vi "测试报告_表格.vi"() -> ()   [LabVIEW 2010]
uses:
  <vilib>/Utility/NIReport.llb/NI_report.lvclass
  全局量/自动测试结果.vi
  <vilib>/Utility/NIReport.llb/Append Report Text (str wrap).vi
panel:
  out "XY图":cluster{"Y":dbl[], "Y":dbl[]}[](graph)
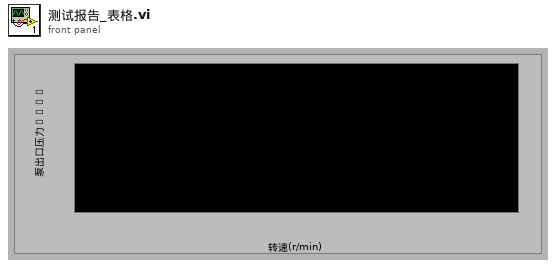
[diagram p1: front panel]
types:
  T1 = enum16{"maximized", "minimized", "normal", "no change"}
  T2 = enum16{"Standard Report", "HTML", "Word", "Excel"}
  T3 = cluster{"position (excel)":cluster{"row":i32, "column":i32}, "name (excel)":string, string}
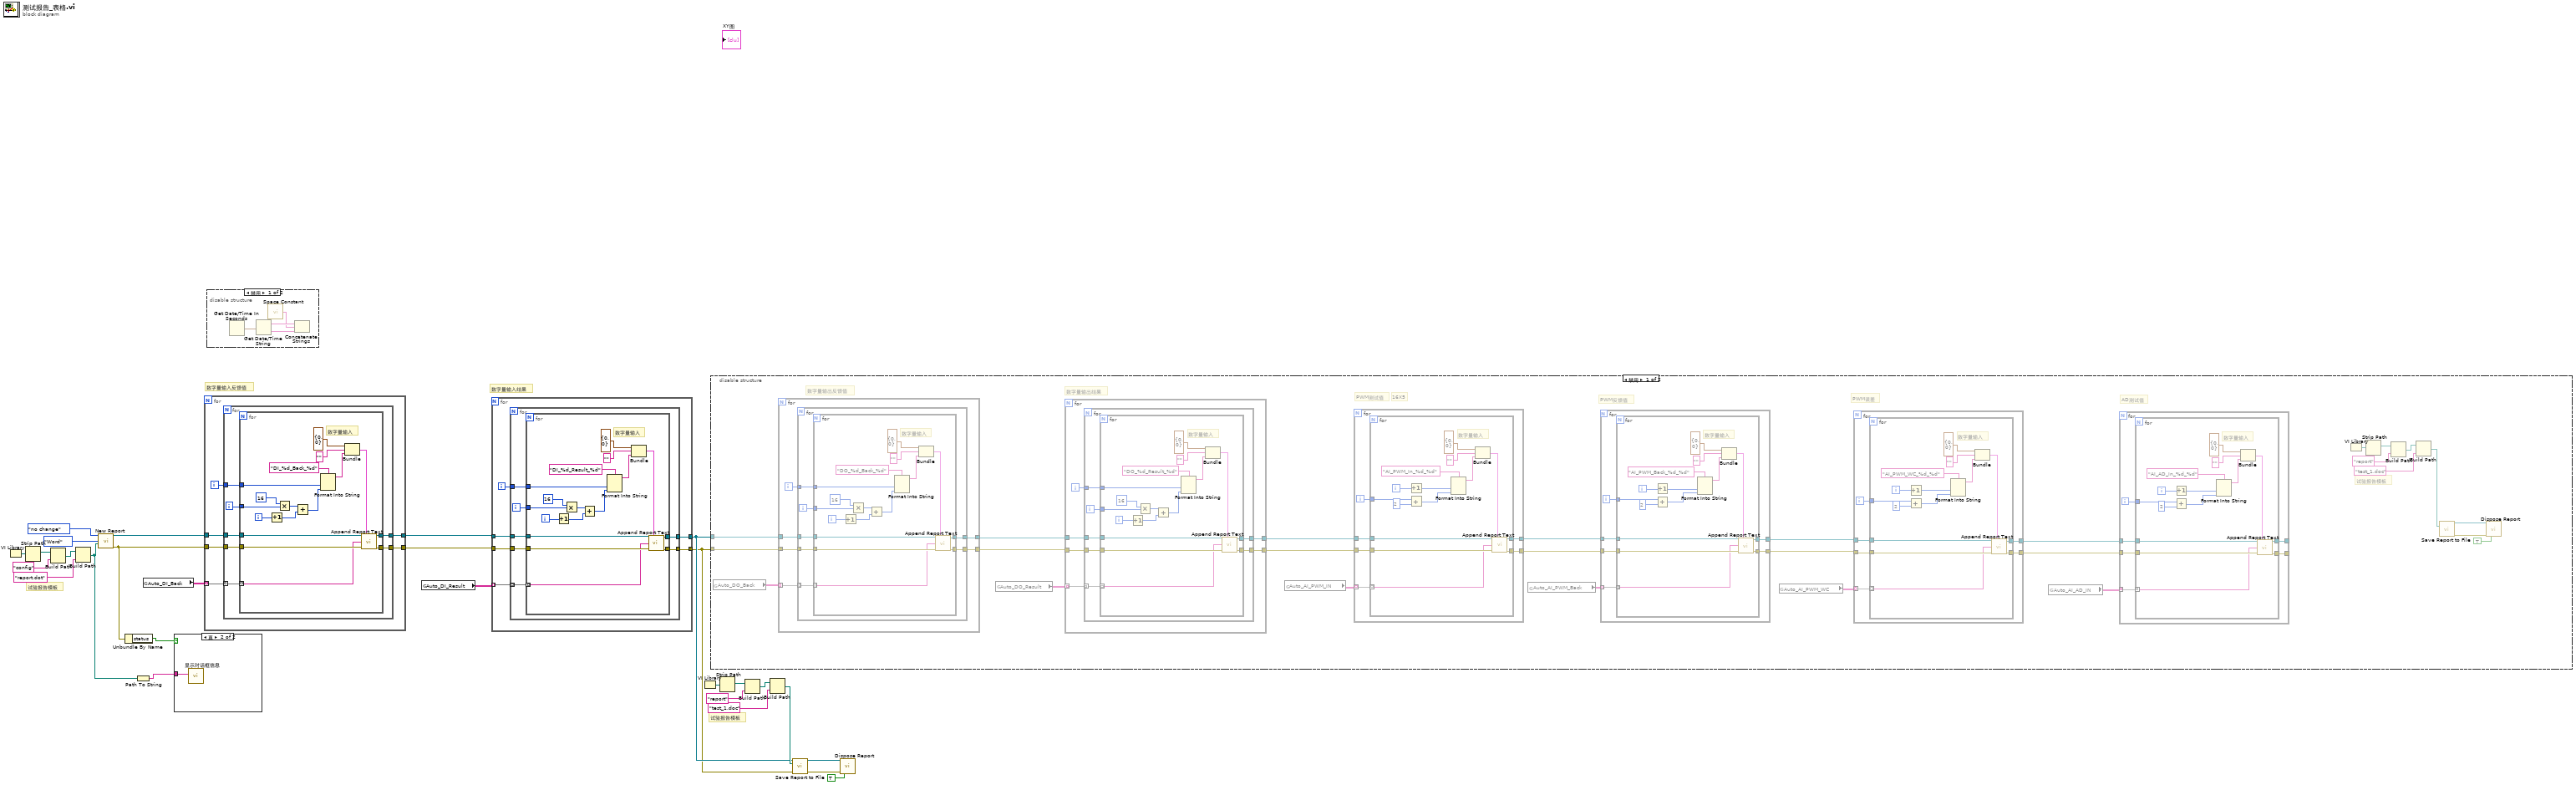
[diagram p0: block diagram]
diagram:
  # "试验报告模板"
  # "数字量输入结果"
  # "数字量输入反馈值"
  # "试验报告模板"
  n1 = VI Library() -> (path=w23:path)
  n2 = Strip Path(path=w23) -> (stripped path=w26:path)  [unwired: 1 out]
  n3 = Build Path(base path=w26, name or relative path="config") -> (appended path=w24:path)
  n4 = Build Path(base path=w24, name or relative path="report.dot") -> (appended path=w2:path)
  n5 = call <vilib>:"New Report.vi"("window state (normal)"=T1."no change", "report type"=T2."Word", "template (empty)"=w2) -> ("report out"=w21:refnum<class "NI_report.lvclass">, "error out"=w5:errorcluster)  [unwired: 11 in]
  n6 = Unbundle By Name(w5) -> ("status"=w4:bool)
  n7 = Path To String(path=w2) -> (string=w1:string)
  n8 = global read "自动测试结果.vi" "Auto_DI_Back"() -> (w20:string[][][])
  n9 = case shown="真" w4 {
    tunnel: w1 -> [_ w28]
    frame False {
    }
    frame True {
      n10 = call "显示对话框信息"("Message"=w28) -> ()  [unwired: 9 in, 2 out]
    }
  }
  n11 = for {
    tunnel: w21 -> [w34]
    tunnel: w5 -> [w33]
    tunnel: [w32] -> w19
    tunnel: [w31] -> w18
    tunnel: w20 -> [w30] mode=indexing
    i -> [w29]
    n12 = for {
      tunnel: w34 -> [w41]
      tunnel: w33 -> [w40]
      tunnel: [w39] -> w32
      tunnel: [w38] -> w31
      tunnel: w30 -> [w36] mode=indexing
      tunnel: w29 -> [w35]
      i -> [w37]
      n13 = for {
        tunnel: w41 -> [w58]
        tunnel: w40 -> [w57]
        tunnel: [w55] -> w39
        tunnel: [w54] -> w38
        tunnel: w37 -> [w46]
        tunnel: w36 -> [w44] mode=indexing
        tunnel: w35 -> [w43]
        i -> [w45]
        # "数字量输入"
        n14 = Increment(x=w45) -> (x+1=w47:i32)
        n15 = Multiply(x=16, y=w46) -> (x*y=w48:i32)
        n16 = Add(x=w48, y=w47) -> (x+y=w42:i32)
        n17 = Format Into String(format string="DI_%d_Back_%d" ("bookmark (word)"), w43, w42) -> (resulting string=w51:string)  [unwired: 2 in, 1 out]
        n18 = Bundle("position (excel)"=cluster{"row":i32, "column":i32} {"row"=0, "column"=0}, "name (excel)"="", w51) -> (w50:T3)  [unwired: 1 in]
        n19 = call-poly <vilib>:"Append Report Text.vi"("report in"=w58, "MS Office parameters"=w50, "text"=w44, "error in (no error)"=w57) -> ("report out"=w55:refnum<class "NI_report.lvclass">, "error out"=w54:errorcluster)  [unwired: 8 in, 2 out]
      }
    }
  }
  n20 = disable-structure shown="禁用" {
    frame Disabled {
      n21 = Get Date/Time In Seconds() -> (seconds since 1Jan1904=w62:timestamp)
      n22 = Get Date/Time String(seconds (now)=w62) -> (date string=w61:string, time string=w60:string)  [unwired: 2 in]
      n23 = call <vilib>:"Space Constant.vi"() -> ("String"=w59:string)
      n24 = Concatenate Strings(w61, w59, w60) -> ()  [unwired: 1 out]
    }
    frame Enabled {
    }
  }
  n25 = global read "自动测试结果.vi" "Auto_DI_Result"() -> (w17:string[][][])
  n26 = for {
    tunnel: w19 -> [w68]
    tunnel: w18 -> [w67]
    tunnel: [w66] -> w7
    tunnel: [w65] -> w6
    tunnel: w17 -> [w64] mode=indexing
    i -> [w63]
    n27 = for {
      tunnel: w68 -> [w75]
      tunnel: w67 -> [w74]
      tunnel: [w73] -> w66
      tunnel: [w72] -> w65
      tunnel: w64 -> [w70] mode=indexing
      tunnel: w63 -> [w69]
      i -> [w71]
      n28 = for {
        tunnel: w75 -> [w92]
        tunnel: w74 -> [w91]
        tunnel: [w89] -> w73
        tunnel: [w88] -> w72
        tunnel: w71 -> [w80]
        tunnel: w70 -> [w78] mode=indexing
        tunnel: w69 -> [w77]
        i -> [w79]
        # "数字量输入"
        n29 = Increment(x=w79) -> (x+1=w81:i32)
        n30 = Multiply(x=16, y=w80) -> (x*y=w82:i32)
        n31 = Add(x=w82, y=w81) -> (x+y=w76:i32)
        n32 = Format Into String(format string="DI_%d_Result_%d" ("bookmark (word)"), w77, w76) -> (resulting string=w85:string)  [unwired: 2 in, 1 out]
        n33 = Bundle("position (excel)"=cluster{"row":i32, "column":i32} {"row"=0, "column"=0}, "name (excel)"="", w85) -> (w84:T3)  [unwired: 1 in]
        n34 = call-poly <vilib>:"Append Report Text.vi"("report in"=w92, "MS Office parameters"=w84, "text"=w78, "error in (no error)"=w91) -> ("report out"=w89:refnum<class "NI_report.lvclass">, "error out"=w88:errorcluster)  [unwired: 8 in, 2 out]
      }
    }
  }
  n35 = VI Library() -> (path=w8:path)
  n36 = disable-structure shown="禁用" {
    disable-tunnel: w7 -> [w110 _]
    disable-tunnel: w6 -> [w109 _]
    frame Disabled {
      # "AD测试值"
      # "PWM误差"
      # "PWM反馈值"
      # "16X5"
      # "PWM测试值"
      # "数字量输出结果"
      # "数字量输出反馈值"
      # "试验报告模板"
      n37 = global read "自动测试结果.vi" "Auto_DO_Back"() -> (w108:string[][][])
      n38 = for {
        tunnel: w110 -> [w239]
        tunnel: w109 -> [w238]
        tunnel: [w237] -> w106
        tunnel: [w236] -> w105
        tunnel: w108 -> [w235] mode=indexing
        i -> [w234]
        n39 = for {
          tunnel: w239 -> [w246]
          tunnel: w238 -> [w245]
          tunnel: [w244] -> w237
          tunnel: [w243] -> w236
          tunnel: w235 -> [w241] mode=indexing
          tunnel: w234 -> [w240]
          i -> [w242]
          n40 = for {
            tunnel: w246 -> [w263]
            tunnel: w245 -> [w262]
            tunnel: [w260] -> w244
            tunnel: [w259] -> w243
            tunnel: w242 -> [w251]
            tunnel: w241 -> [w249] mode=indexing
            tunnel: w240 -> [w248]
            i -> [w250]
            # "数字量输入"
            n41 = Increment(x=w250) -> (x+1=w252:i32)
            n42 = Multiply(x=16, y=w251) -> (x*y=w253:i32)
            n43 = Add(x=w253, y=w252) -> (x+y=w247:i32)
            n44 = Format Into String(format string="DO_%d_Back_%d" ("bookmark (word)"), w248, w247) -> (resulting string=w256:string)  [unwired: 2 in, 1 out]
            n45 = Bundle("position (excel)"=cluster{"row":i32, "column":i32} {"row"=0, "column"=0}, "name (excel)"="", w256) -> (w255:T3)  [unwired: 1 in]
            n46 = call-poly <vilib>:"Append Report Text.vi"("report in"=w263, "MS Office parameters"=w255, "text"=w249, "error in (no error)"=w262) -> ("report out"=w260:refnum<class "NI_report.lvclass">, "error out"=w259:errorcluster)  [unwired: 8 in, 2 out]
          }
        }
      }
      n47 = global read "自动测试结果.vi" "Auto_DO_Result"() -> (w107:string[][][])
      n48 = for {
        tunnel: w106 -> [w209]
        tunnel: w105 -> [w208]
        tunnel: [w207] -> w103
        tunnel: [w206] -> w102
        tunnel: w107 -> [w205] mode=indexing
        i -> [w204]
        n49 = for {
          tunnel: w209 -> [w216]
          tunnel: w208 -> [w215]
          tunnel: [w214] -> w207
          tunnel: [w213] -> w206
          tunnel: w205 -> [w211] mode=indexing
          tunnel: w204 -> [w210]
          i -> [w212]
          n50 = for {
            tunnel: w216 -> [w233]
            tunnel: w215 -> [w232]
            tunnel: [w230] -> w214
            tunnel: [w229] -> w213
            tunnel: w212 -> [w221]
            tunnel: w211 -> [w219] mode=indexing
            tunnel: w210 -> [w218]
            i -> [w220]
            # "数字量输入"
            n51 = Increment(x=w220) -> (x+1=w222:i32)
            n52 = Multiply(x=16, y=w221) -> (x*y=w223:i32)
            n53 = Add(x=w223, y=w222) -> (x+y=w217:i32)
            n54 = Format Into String(format string="DO_%d_Result_%d" ("bookmark (word)"), w218, w217) -> (resulting string=w226:string)  [unwired: 2 in, 1 out]
            n55 = Bundle("position (excel)"=cluster{"row":i32, "column":i32} {"row"=0, "column"=0}, "name (excel)"="", w226) -> (w225:T3)  [unwired: 1 in]
            n56 = call-poly <vilib>:"Append Report Text.vi"("report in"=w233, "MS Office parameters"=w225, "text"=w219, "error in (no error)"=w232) -> ("report out"=w230:refnum<class "NI_report.lvclass">, "error out"=w229:errorcluster)  [unwired: 8 in, 2 out]
          }
        }
      }
      n57 = global read "自动测试结果.vi" "Auto_AI_PWM_IN"() -> (w104:string[][])
      n58 = for {
        tunnel: w103 -> [w188]
        tunnel: w102 -> [w187]
        tunnel: [w186] -> w100
        tunnel: [w185] -> w99
        tunnel: w104 -> [w184] mode=indexing
        i -> [w183]
        n59 = for {
          tunnel: w188 -> [w203]
          tunnel: w187 -> [w202]
          tunnel: [w200] -> w186
          tunnel: [w199] -> w185
          tunnel: w184 -> [w194] mode=indexing
          tunnel: w183 -> [w191]
          i -> [w193]
          # "数字量输入"
          n60 = Increment(x=w193) -> (x+1=w192:i32)
          n61 = Add(x=w191, y=2) -> (x+y=w189:i32)
          n62 = Format Into String(format string="AI_PWM_In_%d_%d" ("bookmark (word)"), w192, w189) -> (resulting string=w196:string)  [unwired: 2 in, 1 out]
          n63 = Bundle("position (excel)"=cluster{"row":i32, "column":i32} {"row"=0, "column"=0}, "name (excel)"="", w196) -> (w195:T3)  [unwired: 1 in]
          n64 = call-poly <vilib>:"Append Report Text.vi"("report in"=w203, "MS Office parameters"=w195, "text"=w194, "error in (no error)"=w202) -> ("report out"=w200:refnum<class "NI_report.lvclass">, "error out"=w199:errorcluster)  [unwired: 8 in, 2 out]
        }
      }
      n65 = global read "自动测试结果.vi" "Auto_AI_PWM_Back"() -> (w101:string[][])
      n66 = for {
        tunnel: w100 -> [w167]
        tunnel: w99 -> [w166]
        tunnel: [w165] -> w97
        tunnel: [w164] -> w96
        tunnel: w101 -> [w163] mode=indexing
        i -> [w162]
        n67 = for {
          tunnel: w167 -> [w182]
          tunnel: w166 -> [w181]
          tunnel: [w179] -> w165
          tunnel: [w178] -> w164
          tunnel: w163 -> [w173] mode=indexing
          tunnel: w162 -> [w170]
          i -> [w172]
          # "数字量输入"
          n68 = Increment(x=w172) -> (x+1=w171:i32)
          n69 = Add(x=w170, y=2) -> (x+y=w168:i32)
          n70 = Format Into String(format string="AI_PWM_Back_%d_%d" ("bookmark (word)"), w171, w168) -> (resulting string=w175:string)  [unwired: 2 in, 1 out]
          n71 = Bundle("position (excel)"=cluster{"row":i32, "column":i32} {"row"=0, "column"=0}, "name (excel)"="", w175) -> (w174:T3)  [unwired: 1 in]
          n72 = call-poly <vilib>:"Append Report Text.vi"("report in"=w182, "MS Office parameters"=w174, "text"=w173, "error in (no error)"=w181) -> ("report out"=w179:refnum<class "NI_report.lvclass">, "error out"=w178:errorcluster)  [unwired: 8 in, 2 out]
        }
      }
      n73 = global read "自动测试结果.vi" "Auto_AI_PWM_WC"() -> (w98:string[][])
      n74 = for {
        tunnel: w97 -> [w146]
        tunnel: w96 -> [w145]
        tunnel: [w144] -> w95
        tunnel: [w143] -> w94
        tunnel: w98 -> [w141] mode=indexing
        i -> [w142]
        n75 = for {
          tunnel: w146 -> [w161]
          tunnel: w145 -> [w160]
          tunnel: [w158] -> w144
          tunnel: [w157] -> w143
          tunnel: w141 -> [w152] mode=indexing
          tunnel: w142 -> [w149]
          i -> [w151]
          # "数字量输入"
          n76 = Increment(x=w151) -> (x+1=w150:i32)
          n77 = Add(x=w149, y=2) -> (x+y=w147:i32)
          n78 = Format Into String(format string="AI_PWM_WC_%d_%d" ("bookmark (word)"), w150, w147) -> (resulting string=w154:string)  [unwired: 2 in, 1 out]
          n79 = Bundle("position (excel)"=cluster{"row":i32, "column":i32} {"row"=0, "column"=0}, "name (excel)"="", w154) -> (w153:T3)  [unwired: 1 in]
          n80 = call-poly <vilib>:"Append Report Text.vi"("report in"=w161, "MS Office parameters"=w153, "text"=w152, "error in (no error)"=w160) -> ("report out"=w158:refnum<class "NI_report.lvclass">, "error out"=w157:errorcluster)  [unwired: 8 in, 2 out]
        }
      }
      n81 = global read "自动测试结果.vi" "Auto_AI_AD_IN"() -> (w93:string[][])
      n82 = for {
        tunnel: w95 -> [w125]
        tunnel: w94 -> [w124]
        tunnel: [w123] -> _
        tunnel: [w122] -> _
        tunnel: w93 -> [w120] mode=indexing
        i -> [w121]
        n83 = for {
          tunnel: w125 -> [w140]
          tunnel: w124 -> [w139]
          tunnel: [w137] -> w123
          tunnel: [w136] -> w122
          tunnel: w120 -> [w131] mode=indexing
          tunnel: w121 -> [w128]
          i -> [w130]
          # "数字量输入"
          n84 = Increment(x=w130) -> (x+1=w129:i32)
          n85 = Add(x=w128, y=2) -> (x+y=w126:i32)
          n86 = Format Into String(format string="AI_AD_In_%d_%d" ("bookmark (word)"), w129, w126) -> (resulting string=w133:string)  [unwired: 2 in, 1 out]
          n87 = Bundle("position (excel)"=cluster{"row":i32, "column":i32} {"row"=0, "column"=0}, "name (excel)"="", w133) -> (w132:T3)  [unwired: 1 in]
          n88 = call-poly <vilib>:"Append Report Text.vi"("report in"=w140, "MS Office parameters"=w132, "text"=w131, "error in (no error)"=w139) -> ("report out"=w137:refnum<class "NI_report.lvclass">, "error out"=w136:errorcluster)  [unwired: 8 in, 2 out]
        }
      }
      n89 = VI Library() -> (path=w119:path)
      n90 = Strip Path(path=w119) -> (stripped path=w116:path)  [unwired: 1 out]
      n91 = Build Path(base path=w116, name or relative path="report") -> (appended path=w118:path)
      n92 = Build Path(base path=w118, name or relative path="test_1.doc") -> (appended path=w114:path)
      n93 = call-dynamic "Save Report to File.vi"("report file path"=w114) -> ("report out"=w113:refnum<class "NI_report.lvclass">, "error out"=w112:errorcluster)  [unwired: 13 in]
      n94 = call-dynamic "Dispose Report.vi"("report in"=w113, "error in (no error)"=w112, "close report? (T)"=TRUE) -> ()  [unwired: 12 in, 1 out]
    }
    frame Enabled {
    }
  }
  n95 = Strip Path(path=w8) -> (stripped path=w11:path)  [unwired: 1 out]
  n96 = Build Path(base path=w11, name or relative path="report") -> (appended path=w9:path)
  n97 = Build Path(base path=w9, name or relative path="test_1.doc") -> (appended path=w13:path)
  n98 = call-dynamic "Save Report to File.vi"("report in"=w7, "report file path"=w13, "error in (no error)"=w6) -> ("report out"=w14:refnum<class "NI_report.lvclass">, "error out"=w15:errorcluster)  [unwired: 11 in]
  n99 = call-dynamic "Dispose Report.vi"("report in"=w14, "error in (no error)"=w15, "close report? (T)"=TRUE) -> ()  [unwired: 12 in, 1 out]
